vi "Ballard - 1553 - Generate Configuration Files.vi"(8 "error in (no error)":errorcluster, 11 "Node Ptr":u64 format="%.0x") -> (0 "error out":errorcluster)   [LabVIEW 2020, in "Ballard 1553 System Explorer.lvlib"]
uses:
  Ballard 1553 System Explorer.lvlib
  Shared/Controls and Global/Global.vi
  <vilib>/NI VeriStand/Custom Device API/Get Item Property (Path).vi
  <vilib>/NI VeriStand/Custom Device API/Custom Device API.lvlib
  Shared/Ballard 1553 Shared.lvlib
panel:
  in  "Tag":string
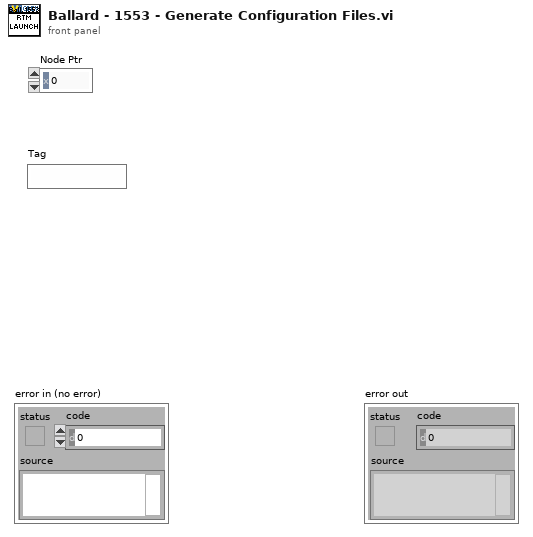
[diagram p1: front panel]
types:
  T1 = typedef "Custom Device API.lvlib/Custom Device Item Ref.ctl" = u64
  T2 = typedef "result_type.ctl" = cluster{"Hw configuration out":path, "Param configuration out":path, "successful generation":bool}
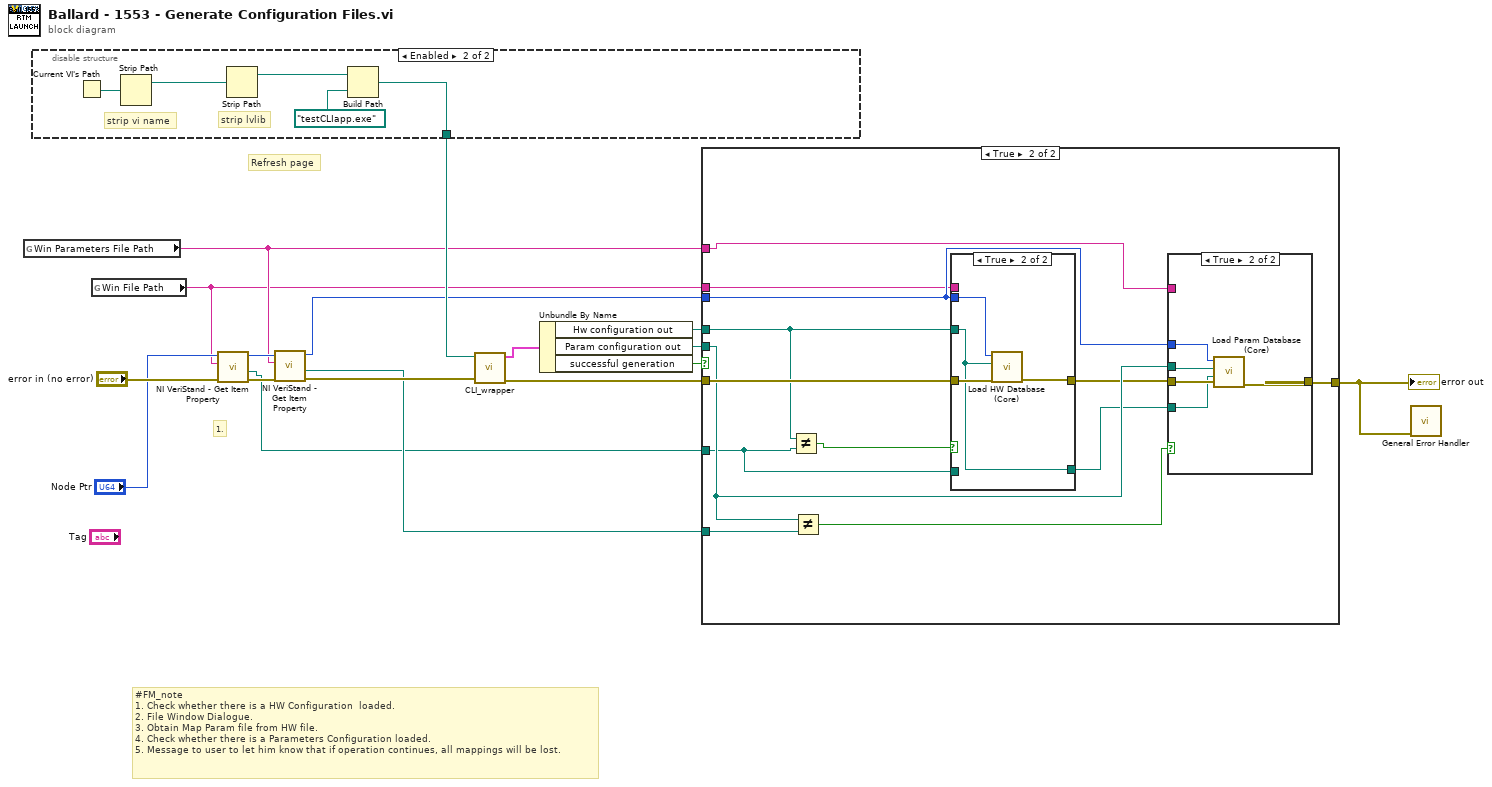
[diagram p0: block diagram]
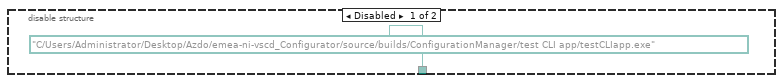
[diagram p2: hidden frame]
diagram:
  # "Refresh page"
  # "#FM_note \n1. Check whether there is a HW Configuration  loaded.\n2. File Window Dialogue.\n3. Obtain Map Param file from HW file.\n4. Check whether there is a Parameters Configuration loaded.\n5. Message to user to let him know that if operation continues, all mappings will be lost."
  # "1."
  n1 = global read "Global.vi" "Win Parameters File Path"() -> (w6:string)
  n2 = disable-structure shown="Enabled" {
    disable-tunnel: [path "C:/Users/Administrator/Desktop/Azdo/emea-ni-vscd_Configurator/source/builds/ConfigurationManager/test CLI app/testCLIapp.exe" ("exe") w19] -> w8
    frame Disabled {
    }
    frame Enabled {
      # "strip lvlib"
      # "strip vi name"
      n3 = Current VI's Path() -> (path=w23:path)
      n4 = Strip Path(path=w23) -> (stripped path=w22:path)  [unwired: 1 out]
      n5 = Strip Path(path=w22) -> (stripped path=w21:path)  [unwired: 1 out]
      n6 = Build Path(base path=w21, name or relative path=path "testCLIapp.exe") -> (appended path=w19:path)
    }
  }
  n7 = global read "Global.vi" "Win File Path"() -> (w5:string)
  n8 = call-poly <vilib>:"NI VeriStand - Get Item Property.vi"("error in (no error)"="error in (no error)", "Property Name"=w5, "Item Ref in"="Node Ptr") -> ("error out"=w15:errorcluster, "Value"=w1:path, "Item Ref out"=w14:T1)  [unwired: 5 in, 1 out]
  n9 = call-poly <vilib>:"NI VeriStand - Get Item Property.vi"("error in (no error)"=w15, "Property Name"=w6, "Item Ref in"=w14) -> ("error out"=w13:errorcluster, "Value"=w2:path, "Item Ref out"=w3:T1)  [unwired: 5 in, 1 out]
  n10 = call "CLI_wrapper.vi"("error in"=w13, "exe"=w8) -> ("error out"=w12:errorcluster, "result"=w11:T2)  [unwired: 8 in]
  n11 = Unbundle By Name(w11) -> ("Hw configuration out"=w7:path, "Param configuration out"=w9:path, "successful generation"=w10:bool)
  n12 = case shown="True" w10 {
    tunnel: [w24 w32] -> w4
    tunnel: w12 -> [w24 w37]
    tunnel: w9 -> [_ w28]
    tunnel: w7 -> [_ w34]
    tunnel: w6 -> [_ w31]
    tunnel: w5 -> [_ w33]
    tunnel: w3 -> [_ w36]
    tunnel: w2 -> [_ w30]
    tunnel: w1 -> [_ w26]
    frame False {
    }
    frame True {
      n13 = Not Equal?(x=w34, y=w26) -> (x != y?=w35:bool)
      n14 = Not Equal?(x=w28, y=w30) -> (x != y?=w29:bool)
      n15 = case shown="True" w35 {
        tunnel: w37 -> [w39 w43]
        tunnel: w36 -> [_ w41]
        tunnel: w34 -> [_ w40]
        tunnel: [w39 w42] -> w27
        tunnel: w33 -> [_ _]
        tunnel: w26 -> [w38 _]
        tunnel: [w38 w40] -> w25
        frame False {
        }
        frame True {
          n16 = call "Load HW Database (Core).vi"("error in"=w43, "hw db path in"=w40, "Node Ptr"=w41) -> ("error out"=w42:errorcluster)  [unwired: 8 in]
        }
      }
      n17 = case shown="True" w29 {
        tunnel: w27 -> [w44 w49]
        tunnel: w36 -> [_ w48]
        tunnel: w28 -> [_ w47]
        tunnel: [w44 w45] -> w32
        tunnel: w31 -> [_ _]
        tunnel: w25 -> [_ w46]
        frame False {
        }
        frame True {
          n18 = call "Load Param Database (Core).vi"("error in"=w49, "hw db path in"=w46, "parm db path in"=w47, "Node Ptr"=w48) -> ("error out"=w45:errorcluster)  [unwired: 7 in]
        }
      }
    }
  }
  "error out" <- w4
  n19 = call <vilib>:"General Error Handler.vi"("error in (no error)"=w4) -> ()  [unwired: 10 in, 5 out]
